vi "Pneumatic Control Controller.vi"(8 "error in":errorcluster) -> ()   [LabVIEW 2016]
doc: "This VI executes continuously carrying out the current operation and responding to updates or new operations. It will often contain the timing or control code that is difficult to place directly in TeleOp. This VI generally opens all sensors and motors and isolates the rest of the robot code from knowing how the operations are carried out."
uses:
  Pneumatic Control Setpoints.ctl
  Pneumatic Control Operations.ctl
  <vilib>/Rock Robotics/WPI/AnalogOutput/WPI_AnalogOutputChannel.ctl
  <vilib>/Rock Robotics/Network Tables/NT Write Boolean.vi
panel:
  in  "NavX Ch 0 Voltage":dbl=5.0 min=0.0 max=5.0
  out "Current\nCmd":string
  # "Tip: It may be helpful to observe inputs and sensor values.\nYou may also want to display tuning or debugging controls."
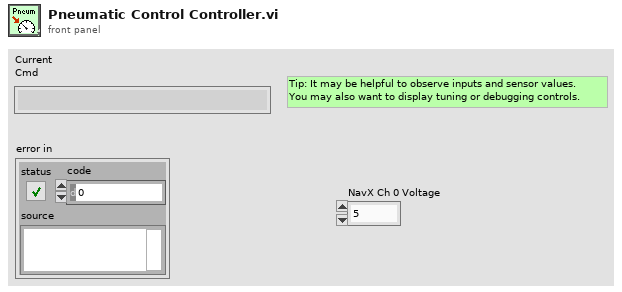
[diagram p1: front panel]
types:
  T1 = typedef "Pneumatic Control Setpoints.ctl" = cluster{"Operation":T2, "Setpoint":dbl, "Duration":dbl}
  T2 = typedef "Pneumatic Control Operations.ctl" = enum16{"Reserve", "Read Current", "Immediate"}
  T3 = typedef "Command Status Info.ctl" = cluster{"Name":string, "Status":T4, "notifier out":T5}
  T4 = typedef "Completion Status.ctl" = enum16{"Successful", "Aborted", "Incomplete"}
  T5 = typedef "Completion Notifier.ctl" = refnum<notifier>
  T6 = cluster{"Default Command":T1, "Command Timing":cluster{"Start Time (ms)":u32, "Iterations":i32}, "Command Arguments":cluster{"Command Info":T3, "Description":string, "Default Command":T1, "notifier out":refnum<notifier>, "Subsystem Name":string}}
  T7 = typedef "WPI_AnalogOutputChannel.ctl" = enum8{"AO MXP 0", "AO MXP 1", "Invalid"}
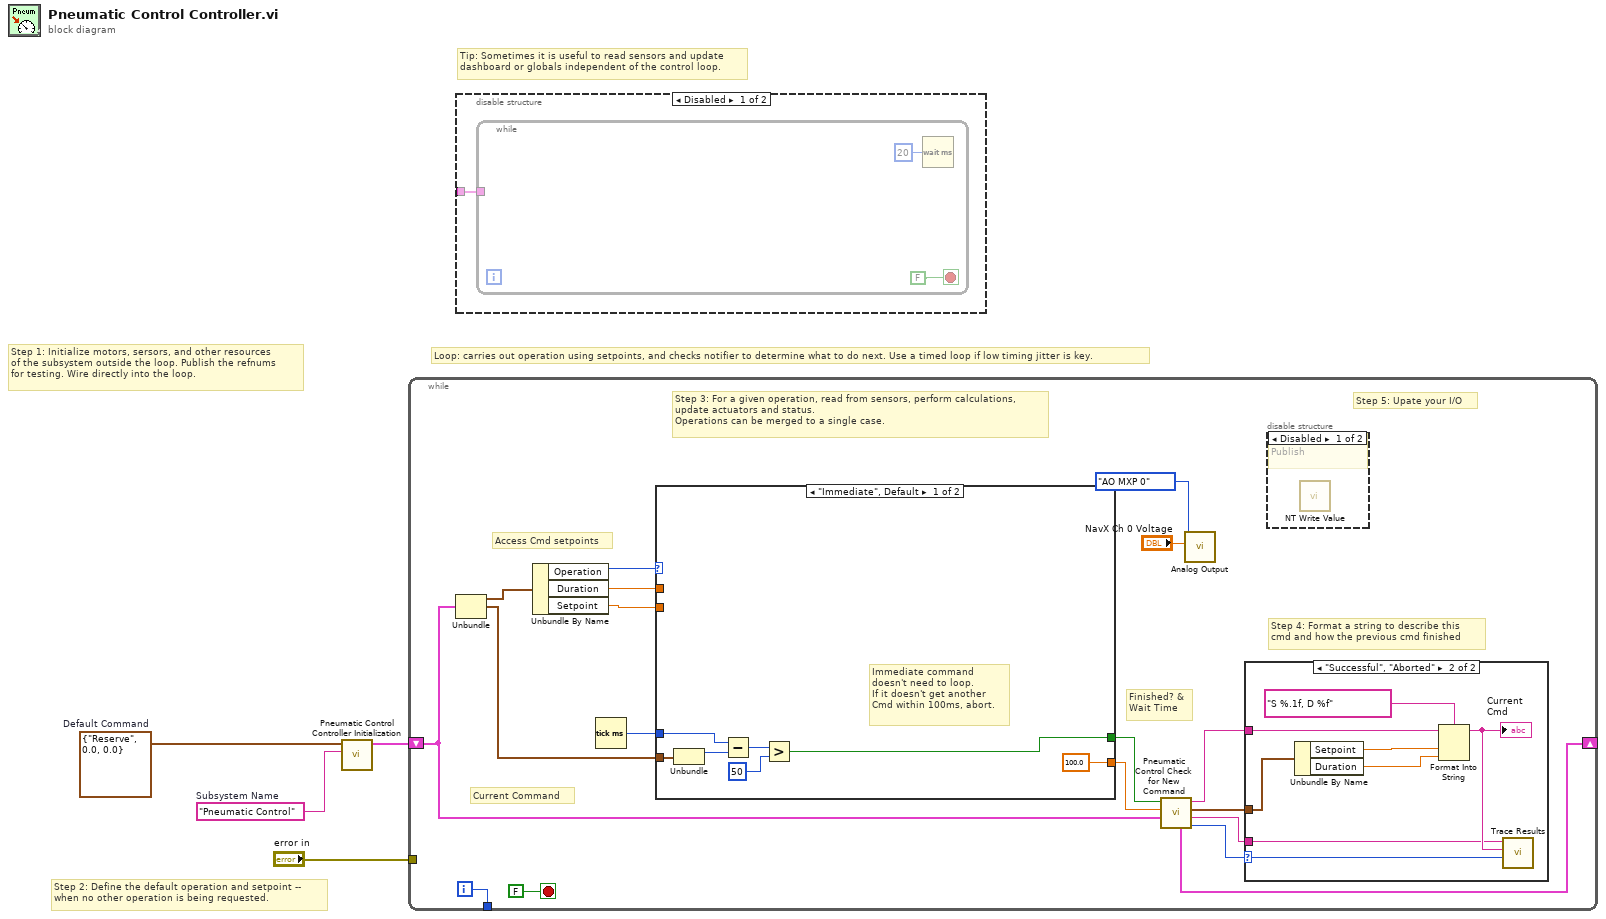
[diagram p0: block diagram]
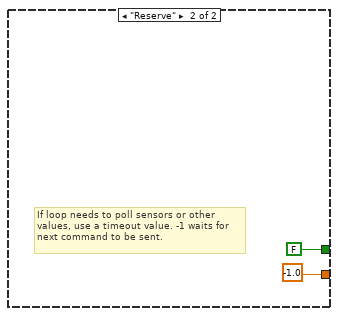
[diagram p5: hidden frame]
diagram:
  w1 = T1 {"Operation"=enum."Reserve", "Setpoint"=0.0, "Duration"=0.0}  # Default Command
  w2 = "Pneumatic Control"  # Subsystem Name
  # "Tip: Sometimes it is useful to read sensors and update\ndashboard or globals independent of the control loop."
  # "Step 2: Define the default operation and setpoint --\nwhen no other operation is being requested."
  # "Step 1: Initialize motors, sersors, and other resources\nof the subsystem outside the loop. Publish the refnums\nfor testing. Wire directly into the loop."
  # "Loop: carries out operation using setpoints, and checks notifier to determine what to do next. Use a timed loop if low timing jitter is key."
  n1 = call "Pneumatic Control Controller Initialization.vi"("Subsystem Name"=w2, "Default Command"=w1) -> ("Command Info"=w3:T6)  [unwired: 9 in]
  n2 = while {
    shift-right: [w13] -> _
    shift-left: w3 -> [w14]
    tunnel: [w21] -> _
    tunnel: "error in" -> [_]
    i -> [w21]
    stop <- FALSE stop-if-true
    # "Step 5: Upate your I/O"
    # "Step 4: Format a string to describe this\ncmd and how the previous cmd finished"
    # "Current Command"
    # "Access Cmd setpoints"
    # "Finished? &\nWait Time"
    # "Step 3: For a given operation, read from sensors, perform calculations,\nupdate actuators and status.\nOperations can be merged to a single case."
    n3 = Unbundle(w14) -> ("Default Command"=w20:T1, "Command Timing"=w16:cluster{"Start Time (ms)":u32, "Iterations":i32})  [unwired: 1 out]
    n4 = Unbundle By Name(w20) -> ("Operation"=w19:T2, "Duration"=w18:dbl, "Setpoint"=w15:dbl)
    n5 = Tick Count (ms)() -> (millisecond timer value=w17:u32)
    n6 = case shown="\"Immediate\", Default" w19 {
      tunnel: [100.0 -1.0] -> w11
      tunnel: [w31 FALSE ("ignore previous (F)")] -> w12
      tunnel: w16 -> [w33 _]
      tunnel: w18 -> [_ _]
      tunnel: w17 -> [w32 _]
      tunnel: w15 -> [_ _]
      frame "Immediate", Default {
        # "Immediate command\ndoesn't need to loop.\nIf it doesn't get another\nCmd within 100ms, abort."
        n7 = Unbundle(w33) -> ("Start Time (ms)"=w36:u32)  [unwired: 1 out]
        n8 = Subtract(x=w32, y=w36) -> (x-y=w35:u32)
        n9 = Greater?(x=w35, y=u8 50 ("Left Motor")) -> (0:w31:bool)
      }
      frame "Reserve" {
        # "If loop needs to poll sensors or other\nvalues, use a timeout value. -1 waits for\nnext command to be sent."
      }
    }
    n10 = call "Pneumatic Control Check for New Command.vi"("Current Command"=w14, "Wait time (ms)"=w11, "Finished?"=w12) -> ("Completion"=w7:T4, "Subsystem Name"=w8:string, "Current Command"=w9:T1, "Initial Trace String"=w10:string, "NextCommand"=w13:T6)  [unwired: 4 in]
    n11 = call <vilib>:"Analog Output.vi"("Voltage"="NavX Ch 0 Voltage", "AO Channel"=WPI_AnalogOutputChannel."AO MXP 0") -> ()  [unwired: 10 in]
    n12 = case shown="\"Successful\", \"Aborted\"" w7 {
      selector: w7 -> [_ w30]
      tunnel: w10 -> [_ w26]
      tunnel: w9 -> [_ w27]
      tunnel: w8 -> [_ w23]
      frame "Incomplete", Default {
        # "Continuing current command"
      }
      frame "Successful", "Aborted" {
        # "Report and setup for next command"
        n13 = Unbundle By Name(w27) -> ("Setpoint"=w29:dbl, "Duration"=w24:dbl)
        n14 = Format Into String(format string="S %.1f, D %f", initial string=w26, w29, w24) -> (resulting string=w25:string)  [unwired: 1 in, 1 out]
        "Current\nCmd" <- w25
        n15 = call <vilib>:"Trace Results.vi"("Status of previous command"=w30, "Description"=w25, "Subsystem"=w23) -> ()  [unwired: 9 in]
      }
    }
    n16 = disable-structure shown="Disabled" {
      frame Disabled {
        # "Publish"
        n17 = call-poly <vilib>:"NT Write Value.vi"() -> ()  [unwired: 11 in, 1 out]
      }
      frame Enabled {
      }
    }
  }
  n18 = disable-structure shown="Disabled" {
    disable-tunnel: _ -> [w40 _]
    frame Disabled {
      n19 = while {
        tunnel: w40 -> [_]
        stop <- FALSE stop-if-true
        n20 = Wait (ms)(milliseconds to wait=u32 20) -> ()  [unwired: 1 out]
      }
    }
    frame Enabled {
    }
  }
